vi "Draw Gate.vi"(4 "error in (no error)":errorcluster, 5 "Upper Limit":dbl, 6 "Lower Limit":dbl, 7 "XYGraph reference":refnum<vi>) -> (0 "error out":errorcluster)   [LabVIEW 2012]
uses:
  <vilib>/Utility/miscctls.llb/LVCursorListTypeDef.ctl
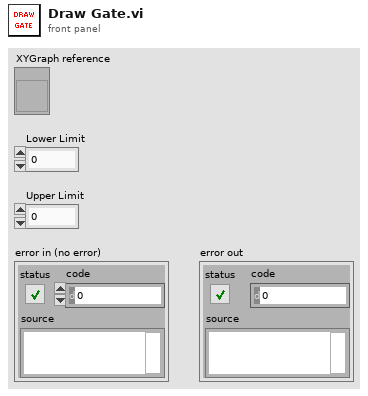
[diagram p1: front panel]
types:
  T1 = typedef "LVCursorListTypeDef.ctl" = cluster{"Name":string, "Color":u32, "Style":u8, "Point Style":u8, "Name Visible":bool, "Allow Drag":bool, "Cursor Mode":u32, "Plot":i32, "Index":i32, "Position":cluster{"X":dbl, "Y":dbl}, "X Scale":u32, "Y Scale":u32, "Watch Plots":i32[], "Watch All Plots":bool, "Plot Area":i32, "Label Offset":cluster{"X":dbl, "Y":dbl}}[]
  T2 = cluster{"Name":string, "Color":u32, "Style":u8, "Point Style":u8, "Name Visible":bool, "Allow Drag":bool, "Cursor Mode":u32, "Plot":i32, "Index":i32, "Position":cluster{"X":dbl, "Y":dbl}, "X Scale":u32, "Y Scale":u32, "Watch Plots":i32[], "Watch All Plots":bool, "Plot Area":i32, "Label Offset":cluster{"X":dbl, "Y":dbl}}
  T3 = cluster{"Name":string, "Color":u32, "Style":u8, "Point Style":u8, "Name Visible":bool, "Allow Drag":bool, "Cursor Mode":u32, "Plot":i32, "Index":i32, "Position":cluster{"X":dbl, "Y":dbl}, "X Scale":u32, "Y Scale":u32, "Watch Plots":i32[], "Watch All Plots":bool, "Plot Area":i32, "Label Offset":cluster{"X":dbl, "Y":dbl}}[]
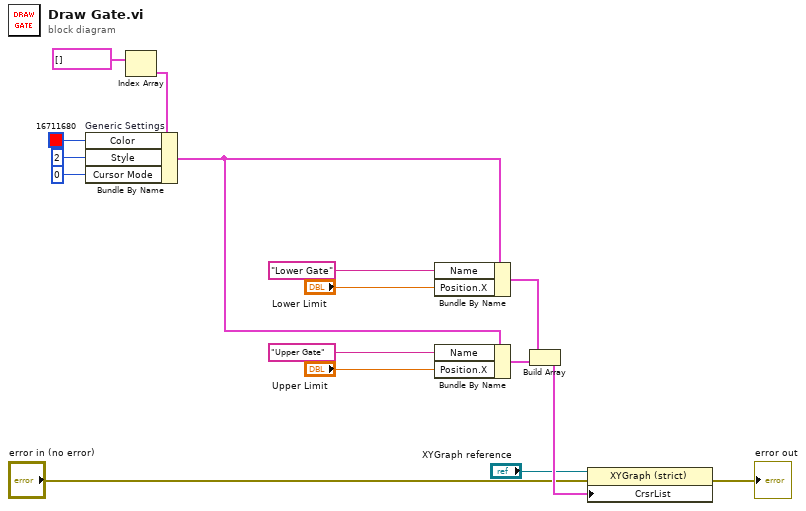
[diagram p0: block diagram]
diagram:
  n1 = Index Array(array=T1 [] ("Cursor List")) -> (element=w5:T2)  [unwired: 1 in]
  n2 = Bundle By Name "Generic Settings"(cluster=w5, "Color"=u32 16711680, "Style"=u8 2, "Cursor Mode"=u32 0) -> (w4:T2)
  n3 = Bundle By Name(cluster=w4, "Name"="Lower Gate", "Position.X"="Lower Limit") -> (w12:T2)
  n4 = Bundle By Name(cluster=w4, "Name"="Upper Gate", "Position.X"="Upper Limit") -> (w9:T2)
  n5 = Build Array(w12, w9) -> (w16:T3)
  n6 = property on="Property Node" class="XYGraph (strict)"(reference="XYGraph reference", error in="error in (no error)", "CrsrList"=w16) -> (error out=→"error out":errorcluster)  [unwired: 1 out]
